vi "Counter Embedded.vi"(9 "Reset":bool, 10 "Digital Limit":u32, 11 "Digital Count In":u32) -> (2 "Limit Reached":bool, 3 "Digital Count Out":u32)   [LabVIEW 2015]
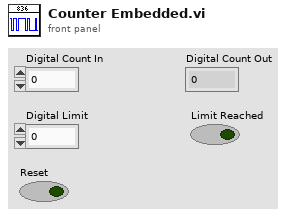
[diagram p1: front panel]
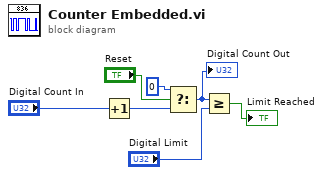
[diagram p0: block diagram]
diagram:
  n1 = Increment(x="Digital Count In") -> (x+1=w3:u32)
  n2 = Select(t=u32 0, s="Reset", f=w3) -> (s? t:f=w4:u32)
  "Digital Count Out" <- w4
  n3 = Greater Or Equal?(x=w4, y="Digital Limit") -> (x >= y?=→"Limit Reached":bool)
